vi "StopRequest.vi"(8 "error in (no error)":errorcluster, 9 "Wait for Module to stop? (F)":bool, 11 "ModuleAdmin":refnum<class "ModuleAdmin.lvclass">) -> (0 "error out":errorcluster, 2 "Wait to Stop":bool, 3 "ModuleAdmin":refnum<class "ModuleAdmin.lvclass">)   [LabVIEW 2018, in "PluginsShared.lvlib"]
doc: "Sends a message to the module to stop operation and close."
uses:
  PluginsShared.lvlib
  <userlib>/NIST/ModuleAdminLib/ModuleAdmin/ModuleAdmin.lvclass
  <vilib>/event_ctls.llb/usereventprio.ctl
  clStopArgument.ctl
  clEventType.ctl
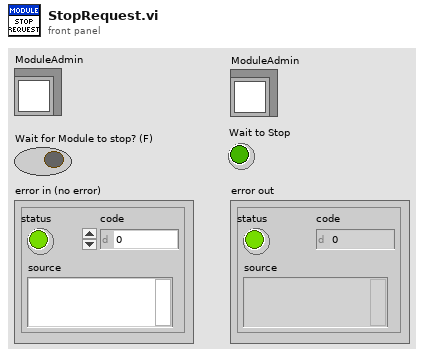
[diagram p1: front panel]
types:
  T1 = typedef "PluginsShared.lvlib/clRequestEvents.ctl" = cluster{"StopRequest":refnum<user-event>, "PathToINI":refnum<user-event>, " LoadPlugin":refnum<user-event>, "ShowPanel":refnum<user-event>, "PrefDlg":refnum<user-event>}
  T2 = typedef "PluginsShared.lvlib/clEventType.ctl" = cluster{"ModuleID":i32, "Data":variant}
  T3 = typedef "PluginsShared.lvlib/clStopArgument.ctl" = cluster{"Exit via Stop Module Req?":bool, "Wait for Module to stop?":bool, "ModuleAdmin":refnum<class "ModuleAdmin.lvclass">}
  T4 = typedef "usereventprio.ctl" = enum32{"high priority", "normal priority"}
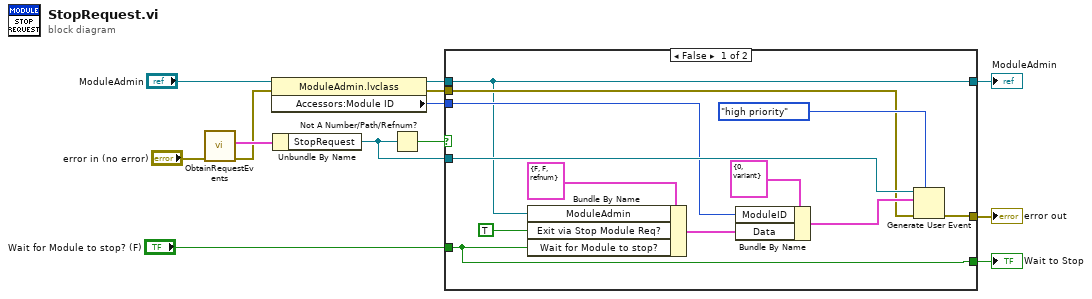
[diagram p0: block diagram]
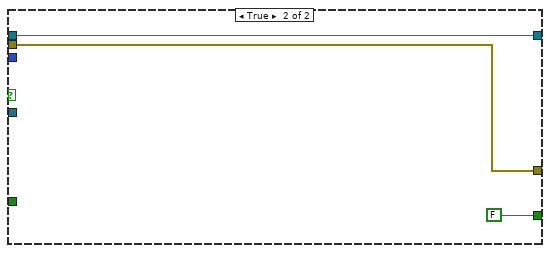
[diagram p2: hidden frame]
diagram:
  n1 = call "ObtainRequestEvents.vi"("error in (no error)"="error in (no error)") -> ("error out"=w2:errorcluster, "clRequestEvents"=w13:T1)  [unwired: 9 in]
  n2 = property class="ModuleAdmin.lvclass"(reference="ModuleAdmin", error in=w2) -> (reference out=w4:refnum<class "ModuleAdmin.lvclass">, error out=w5:errorcluster, "Accessors:Module ID"=w7:i32)
  n3 = Unbundle By Name(w13) -> ("StopRequest"=w11:refnum<user-event>)
  n4 = Not A Number/Path/Refnum?(number/path/refnum=w11) -> (NaN/Path/Refnum?=w12:bool)
  n5 = case shown="False" w12 {
    tunnel: w11 -> [w25 _]
    tunnel: "Wait for Module to stop? (F)" -> [w16 _]
    tunnel: [w18 w27] -> w9
    tunnel: w7 -> [w17 _]
    tunnel: [w16 FALSE] -> w6
    tunnel: w5 -> [w15 w27]
    tunnel: w4 -> [w14 w26]
    tunnel: [w14 w26] -> w1
    frame False {
      n6 = Bundle By Name(cluster=T3 {"Exit via Stop Module Req?"=FALSE, "Wait for Module to stop?"=FALSE, "ModuleAdmin"=refnum} ("Stop Argument"), "ModuleAdmin"=w14, "Exit via Stop Module Req?"=TRUE, "Wait for Module to stop?"=w16) -> (w20:T3)
      n7 = Bundle By Name(cluster=T2 {"ModuleID"=0, "Data"=variant} ("clBroadcast"), "ModuleID"=w17, "Data"=w20) -> (w19:T2)
      n8 = Generate User Event(priority (normal)=usereventprio."high priority", user event=w25, event data cluster=w19, error in=w15) -> (error out=w18:errorcluster)  [unwired: 1 out]
    }
    frame True {
    }
  }
  "error out" <- w9
  "Wait to Stop" <- w6
  "ModuleAdmin" <- w1
